vi "GeneratePoint.vi"(2 "Radius":u32=1, 3 "Offset":sgl min=-360 max=360 step=1 format="%#.0f", 4 "Resolution":u16=360 min=180 max=720 step=180, 5 "Angle":i16=360 min=-360 max=360 step=1) -> (0 "y-disp":sgl[](array[numeric]), 1 "x-disp":sgl[](array[numeric]))   [LabVIEW 2010]
uses:
  <vilib>/express/express arith-compare/Formula/XNode/ExpressFormulaBlockNode.xnode
panel:
  out "Dummy":sgl
  out "Dummy2":dbl
  out "XY Graph":cluster{"Y":dbl[], "Y":dbl[]}[](graph)
  # "Inputs"
  # "Outputs"
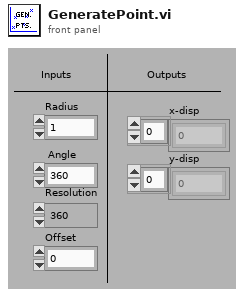
[diagram p1: front panel]
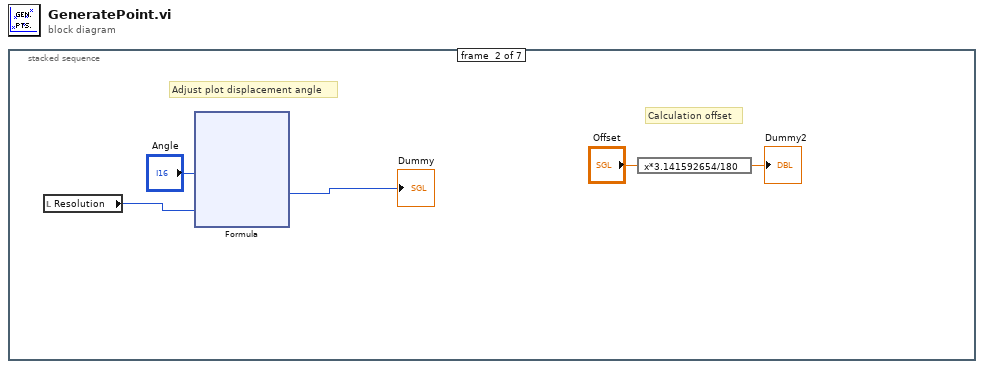
[diagram p0: block diagram]
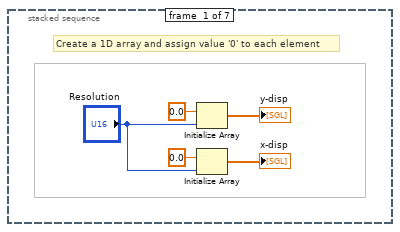
[diagram p2: hidden frame]
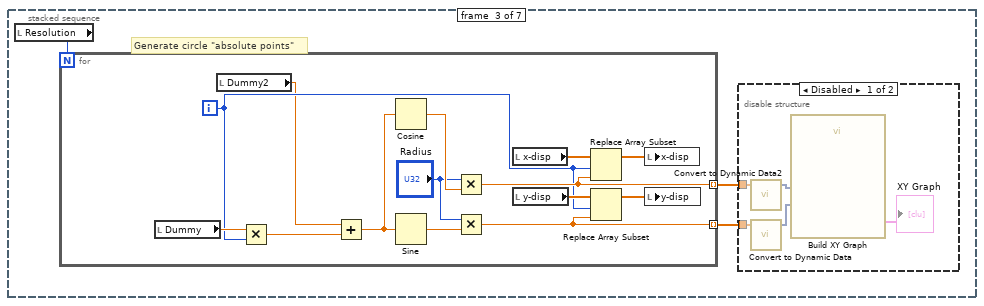
[diagram p3: hidden frame]
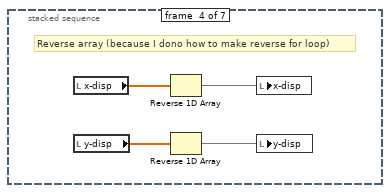
[diagram p5: hidden frame]
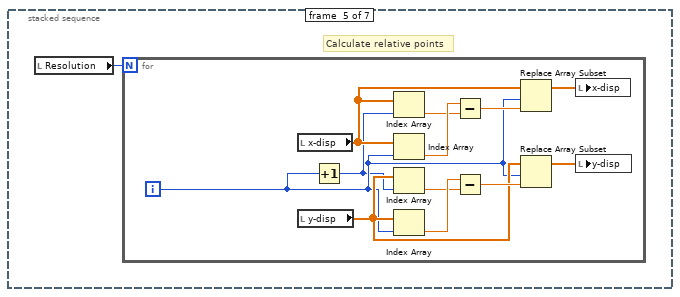
[diagram p6: hidden frame]
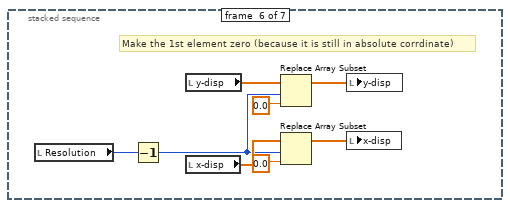
[diagram p7: hidden frame]
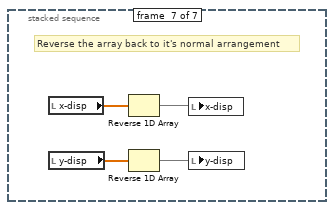
[diagram p8: hidden frame]
diagram:
  n1 = stacked-sequence {
    frame #0 {
      # "Create a 1D array and assign value '0' to each element"
      n2 = Initialize Array(sgl 0.0 ("element"), "Resolution") -> (→"y-disp":sgl[])
      n3 = Initialize Array(sgl 0.0 ("element"), "Resolution") -> (→"x-disp":sgl[])
    }
    frame #1 {
      # "Calculation offset"
      # "Adjust plot displacement angle"
      n4 = local read "Resolution"() -> (w10:u16)
      n5 = xnode "Formula"("X1"="Angle", "X2"=w10) -> ("Result"=→"Dummy":u16)  [unwired: 1 in, 1 out]
      n6 = expression code="x*3.141592654/180"("Offset") -> (→"Dummy2":sgl)
    }
    frame #2 {
      # "Generate circle \"absolute points\""
      n7 = local read "Resolution"() -> (w23:u16)
      n8 = for {
        N: w23 -> [_]
        tunnel: [w34] -> w22 mode=indexing
        tunnel: [w33] -> w21 mode=indexing
        i -> [w32]
        n9 = local read "Dummy"() -> (w40:sgl)
        n10 = local read "Dummy2"() -> (w30:dbl)
        n11 = Multiply(x=w40, y=w32) -> (x*y=w31:sgl)
        n12 = Add(x=w30, y=w31) -> (x+y=w29:dbl)
        n13 = Cosine(x=w29) -> (cos(x)=w39:dbl)
        n14 = Sine(x=w29) -> (sin(x)=w38:dbl)
        n15 = Multiply(x="Radius", y=w39) -> (x*y=w33:dbl)
        n16 = Multiply(x="Radius", y=w38) -> (x*y=w34:dbl)
        n17 = local read "x-disp"() -> (w42:sgl[])
        n18 = local read "y-disp"() -> (w41:sgl[])
        n19 = Replace Array Subset(array=w42, new element=w33, index=w32) -> (w35:sgl[])
        n20 = Replace Array Subset(array=w41, new element=w34, index=w32) -> (w36:sgl[])
        n21 = local write "x-disp"(w35) -> ()
        n22 = local write "y-disp"(w36) -> ()
      }
      n23 = disable-structure shown="Disabled" {
        disable-tunnel: w22 -> [w27 _]
        disable-tunnel: w21 -> [w25 _]
        frame Disabled {
          n24 = call "Convert to Dynamic Data2"("Array"=w25) -> ("Dynamic Data Type"=w24:dynamicdata)  [unwired: 3 in]
          n25 = call "Convert to Dynamic Data"("Array"=w27) -> ("Dynamic Data Type"=w26:dynamicdata)  [unwired: 3 in]
          n26 = call "Build XY Graph"("Y Input"=w26, "X Input"=w24) -> ("XY Graph"=→"XY Graph":cluster{"Y":dbl[], "Y":dbl[]}[])  [unwired: 3 in, 6 out]
        }
        frame Enabled {
        }
      }
    }
    frame #3 {
      # "Reverse array (because I dono how to make reverse for loop)"
      n27 = local read "x-disp"() -> (w46:sgl[])
      n28 = local read "y-disp"() -> (w45:sgl[])
      n29 = Reverse 1D Array(array=w46) -> (reversed array=w44:sgl[])
      n30 = Reverse 1D Array(array=w45) -> (reversed array=w43:sgl[])
      n31 = local write "x-disp"(w44) -> ()
      n32 = local write "y-disp"(w43) -> ()
    }
    frame #4 {
      # "Calculate relative points"
      n33 = local read "Resolution"() -> (w47:u16)
      n34 = for {
        N: w47 -> [_]
        i -> [w49]
        n35 = local read "x-disp"() -> (w53:sgl[])
        n36 = local read "y-disp"() -> (w52:sgl[])
        n37 = Increment(x=w49) -> (x+1=w48:i32)
        n38 = Index Array(array=w53, index=w48) -> (element=w58:sgl)
        n39 = Index Array(array=w53, index=w49) -> (element=w59:sgl)
        n40 = Index Array(array=w52, index=w48) -> (element=w56:sgl)
        n41 = Index Array(array=w52, index=w49) -> (element=w57:sgl)
        n42 = Subtract(x=w59, y=w58) -> (x-y=w55:sgl)
        n43 = Subtract(x=w57, y=w56) -> (x-y=w54:sgl)
        n44 = Replace Array Subset(array=w53, new element=w55, index=w49) -> (w51:sgl[])
        n45 = Replace Array Subset(array=w52, new element=w54, index=w49) -> (w50:sgl[])
        n46 = local write "x-disp"(w51) -> ()
        n47 = local write "y-disp"(w50) -> ()
      }
    }
    frame #5 {
      # "Make the 1st element zero (because it is still in absolute corrdinate)"
      n48 = local read "Resolution"() -> (w61:u16)
      n49 = Decrement(x=w61) -> (x-1=w60:u16)
      n50 = local read "y-disp"() -> (w64:sgl[])
      n51 = local read "x-disp"() -> (w67:sgl[])
      n52 = Replace Array Subset(array=w64, new element=sgl 0.0 ("new element/subarray"), index=w60) -> (w65:sgl[])
      n53 = Replace Array Subset(array=w67, new element=sgl 0.0 ("new element/subarray"), index=w60) -> (w66:sgl[])
      n54 = local write "y-disp"(w65) -> ()
      n55 = local write "x-disp"(w66) -> ()
    }
    frame #6 {
      # "Reverse the array back to it's normal arrangement"
      n56 = local read "x-disp"() -> (w71:sgl[])
      n57 = local read "y-disp"() -> (w68:sgl[])
      n58 = Reverse 1D Array(array=w71) -> (reversed array=w70:sgl[])
      n59 = Reverse 1D Array(array=w68) -> (reversed array=w69:sgl[])
      n60 = local write "x-disp"(w70) -> ()
      n61 = local write "y-disp"(w69) -> ()
    }
  }
